vi "Bluetooth-Server.vi"() -> ()   [LabVIEW 2019]
doc: "Demonstrates how to set up a basic Bluetooth connection, send data to the specified channel once a connection has been established, and terminate the connection once the data has been sent. This VI is designed to stop if the Bluetooth connection is terminated. The data sent in this example is an array of random numbers."
panel:
  in  "Client Closed":string="The client VI closed the connection."
  out "Waveform Graph":dbl[](graph)
  out "Address":string
  out "Channel":u16
  in  "Stop":bool
  # "Overview: Demonstrates the use of the Bluetooth functions to initialize a Bluetooth server that can send data to a client VI.\nRequirements: Bluetooth-enabled computer\nInstructions:\n1. Run the VI.\n2. Open Simple Bluetooth - Client.vi and follow the instructions on its front panel. Note that if you wait longer than 30 seconds to do this after running this VI, it will time out.\n3. Click Stop to stop the VI. Note that if you stop the client VI, this VI will stop automatically."
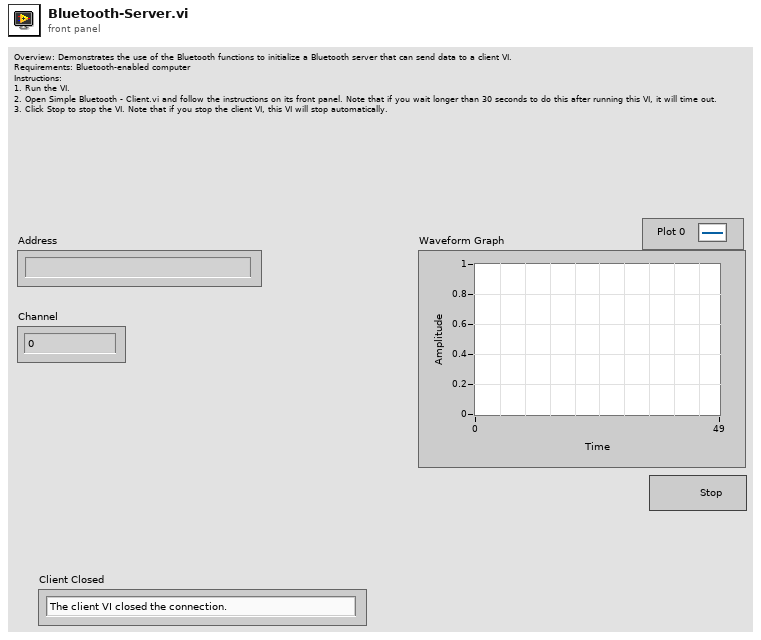
[diagram p1: front panel]
types:
  T1 = cluster{"Address":string, "Device Name":string}[]
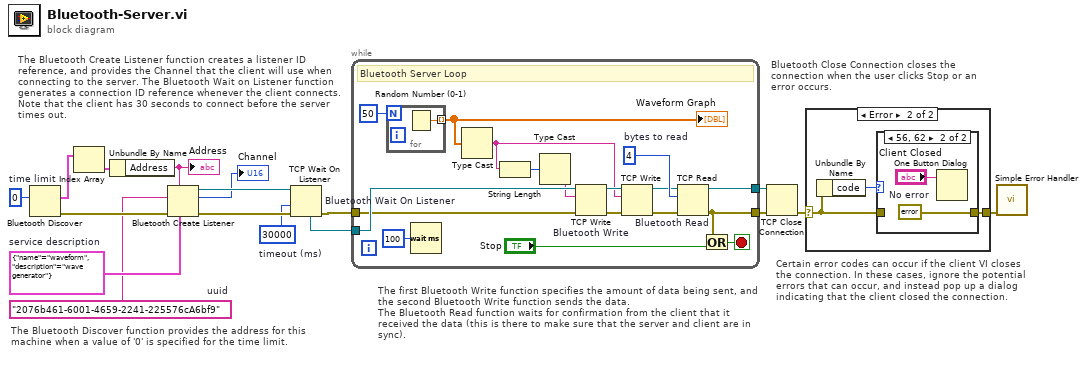
[diagram p0: block diagram]
diagram:
  w6 = cluster{"name":string, "description":string} {"name"="waveform", "description"="wave generator"}  # service description
  w9 = 30000  # timeout (ms)
  w4 = "2076b461-6001-4659-2241-225576cA6bf9"  # uuid
  w12 = 0  # time limit
  # "Bluetooth Close Connection closes the connection when the user clicks Stop or an error occurs."
  # "The Bluetooth Create Listener function creates a listener ID reference, and provides the Channel that the client will use when connecting to the server. The Bluetooth Wait on Listener function generates a connection ID reference whenever the client connects. Note that the client has 30 seconds to connect before the server times out."
  # "The Bluetooth Discover function provides the address for this machine when a value of '0' is specified for the time limit."
  # "Certain error codes can occur if the client VI closes the connection. In these cases, ignore the potential errors that can occur, and instead pop up a dialog indicating that the client closed the connection."
  # "The first Bluetooth Write function specifies the amount of data being sent, and the second Bluetooth Write function sends the data.  \nThe Bluetooth Read function waits for confirmation from the client that it received the data (this is there to make sure that the server and client are in sync)."
  n1 = Bluetooth Discover(10:w12) -> (0:w5:errorcluster, 2:w11:T1)  [unwired: 1 in, 1 out]
  n2 = Index Array(array=w11) -> (element=w10:cluster{"Address":string, "Device Name":string})  [unwired: 1 in]
  n3 = Unbundle By Name(w10) -> ("Address"=w1:string)
  "Address" <- w1
  n4 = Bluetooth Create Listener(6:w6, 7:w1, 8:w5, 10:w4) -> (0:w14:errorcluster, 2:→"Channel":u16, 3:w15:refnum<k31>)
  n5 = TCP Wait On Listener "Bluetooth Wait On Listener"(8:w14, 9:w9, 11:w15) -> (0:w7:errorcluster, 4:w8:refnum<k31>)  [unwired: 4 out]
  n6 = while {
    tunnel: [w18] -> w16
    tunnel: [w19] -> w17
    tunnel: w8 -> [w34]
    tunnel: w7 -> [w25]
    stop <- w27 stop-if-true
    w22 = 4  # bytes to read
    # "Bluetooth Server Loop"
    n7 = for {
      N: 50 ("# of Points") -> [_]
      tunnel: [w35] -> w23 mode=indexing
      n8 = Random Number (0-1)() -> (number: 0 to 1=w35:dbl)
    }
    "Waveform Graph" <- w23
    n9 = Wait (ms)(milliseconds to wait=u32 100) -> ()  [unwired: 1 out]
    n10 = Type Cast(x=w23) -> (*(type *) &x=w29:string)  [unwired: 1 out]
    n11 = String Length(string=w29) -> (length=w31:i32)
    n12 = Type Cast(x=w31) -> (*(type *) &x=w30:string)  [unwired: 1 out]
    n13 = TCP Write "Bluetooth Write"(connection ID=w34, data in=w30, error in (no error)=w25) -> (connection ID out=w33:refnum<k31>, error out=w32:errorcluster)  [unwired: 2 out]
    n14 = TCP Write(connection ID=w33, data in=w29, error in (no error)=w32) -> (connection ID out=w21:refnum<k31>, error out=w20:errorcluster)  [unwired: 2 out]
    n15 = TCP Read "Bluetooth Read"(connection ID=w21, bytes to read=w22, error in (no error)=w20) -> (connection ID out=w19:refnum<k31>, error out=w18:errorcluster)  [unwired: 3 out]
    n16 = Or(x=w18, y="Stop") -> (x .or. y?=w27:bool)
  }
  n17 = TCP Close Connection ("Bluetooth Close Connection")(connection ID=w17, error in (no error)=w16) -> (error out=w3:errorcluster)  [unwired: 2 out]
  n18 = case shown="Error" w3 {
    selector: w3 -> [w36 w38]
    tunnel: [w36 w37] -> w2
    frame No Error {
    }
    frame Error {
      n19 = Unbundle By Name(w38) -> ("code"=w39:i32)
      n20 = case shown="56, 62" w39 {
        tunnel: w38 -> [w40 _]
        tunnel: [w40 w42] -> w37
        frame Default {
        }
        frame 56, 62 {
          w42 = errorcluster {"status"=FALSE, "code"=0, "source"=""}  # No error
          n21 = One Button Dialog(message="Client Closed") -> ()  [unwired: 1 in, 1 out]
        }
      }
    }
  }
  n22 = call <vilib>:"Simple Error Handler.vi"("error in (no error)"=w2) -> ()  [unwired: 1 in, 8 out]
